vi "convert_unit.vi"(0 "input":T2) -> (1 "output":T1, 2 "minus":bool)   [LabVIEW 2013]
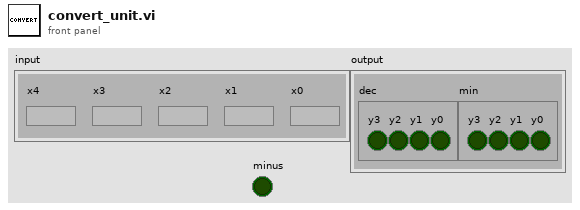
[diagram p1: front panel]
types:
  T1 = cluster{"dec":cluster{"y3":bool, "y2":bool, "y1":bool, "y0":bool}, "min":cluster{"y3":bool, "y2":bool, "y1":bool, "y0":bool}}
  T2 = cluster{"x4":bool, "x3":bool, "x2":bool, "x1":bool, "x0":bool}
  T3 = cluster{"R4":bool, "R3":bool, "R2":bool, bool, "R0":bool}
  T4 = cluster{"min":cluster{"x3":bool, "x2":bool, "x1":bool, "x0":bool}, "dec":cluster{"x3":bool, "x2":bool, "x1":bool, "x0":bool}}
  T5 = cluster{"x3":bool, "x2":bool, "x1":bool, "x0":bool}
  T6 = cluster{"dec":cluster{"x3":bool, "x2":bool, "x1":bool, "x0":bool}, "min":cluster{"x3":bool, "x2":bool, "x1":bool, "x0":bool}}
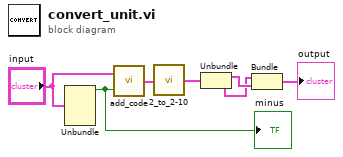
[diagram p0: block diagram]
diagram:
  n1 = Unbundle("input") -> ("x4"=w1:bool)  [unwired: 4 out]
  "minus" <- w1
  n2 = call "add_code.vi"("add_code"=w1, "A"="input") -> ("Result"=w6:T3)
  n3 = call "2_to_2-10.vi"("input"=w6) -> ("output"=w5:T4)
  n4 = Unbundle(w5) -> ("min"=w4:T5, "dec"=w3:T5)
  n5 = Bundle("dec"=w3, "min"=w4) -> (→"output":T6)  [unwired: 1 in]
